vi "SelfTest.vi"(8 "error in (no error)":errorcluster, 11 "Keysight44xx in":refnum<class "Keysight44xx.lvclass">) -> (0 "error out":errorcluster, 1 "SelfTest Message":string, 2 "SelfTestResult":i16, 3 "Keysight44xx out":refnum<class "Keysight44xx.lvclass">)   [LabVIEW 2018, in "SpecAnPlugins.lvlib" / "Keysight44xx.lvclass"]
doc: "This VI runs the instrument's self test routine and returns the test result(s)."
uses:
  Keysight44xx.lvclass
  C:/Users/ico/Documents/Projects/NistPluggableModules/SpecAn/SpecAnPlugins/SpecAnBaseClass/SpecAnBase.lvclass
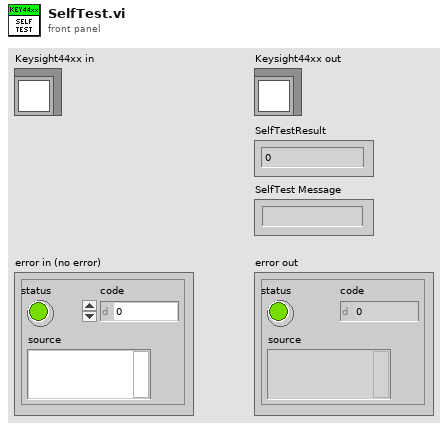
[diagram p1: front panel]
types:
  T1 = typedef "SpecAnPlugins.lvlib/SpecAnBase.lvclass/Acquisition.ctl" = cluster{"Handle":string, "Connected":bool, "Enabled":bool, "SweepModeContinuous":bool, "NumberOfSweeps":i32, "DetectorTypeAuto":bool, "DetectorType":i32, "VerticalScale":i32, "MaximumTime(seconds)":dbl}
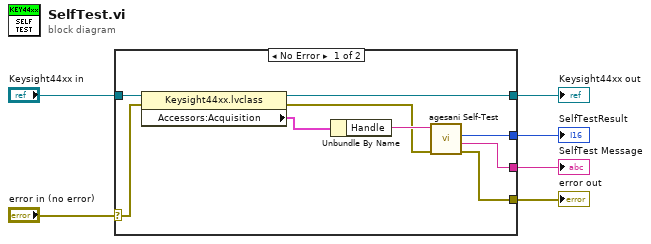
[diagram p0: block diagram]
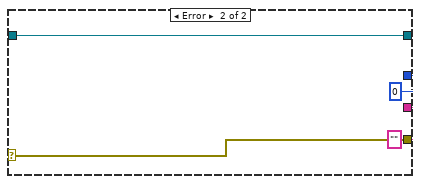
[diagram p2: hidden frame]
diagram:
  n1 = case shown="No Error" "error in (no error)" {
    selector: "error in (no error)" -> [w14 w18]
    tunnel: "Keysight44xx in" -> [w15 w19]
    tunnel: [w10 w19] -> w4
    tunnel: [w9 w18] -> w3
    tunnel: [w8 "" ("self-test message")] -> w2
    tunnel: [w7 i16 0 ("self test result")] -> w1
    frame No Error {
      n2 = property class="Keysight44xx.lvclass"(reference=w15, error in=w14) -> (reference out=w10:refnum<class "Keysight44xx.lvclass">, error out=w11:errorcluster, "Accessors:Acquisition"=w13:T1)
      n3 = Unbundle By Name(w13) -> ("Handle"=w12:string)
      n4 = call <instrlib>:"agesani Self-Test.vi"("error in (no error)"=w11, "instrument handle"=w12) -> ("error out"=w9:errorcluster, "self-test message"=w8:string, "self test result"=w7:i16)  [unwired: 6 in, 1 out]
    }
    frame Error {
    }
  }
  "error out" <- w3
  "Keysight44xx out" <- w4
  "SelfTestResult" <- w1
  "SelfTest Message" <- w2
